vi "Teleop.vi"(10 "Match Info":T3={"Autonomous Elapsed Seconds"=0.0, "TeleOp Elapsed Seconds"=0.0, "Disabled Elapsed Seconds"=0.0, "Visited Autonomous"=FALSE, "Visited TeleOp"=FALSE, "Visited Disabled"=FALSE, "Autonomous Settings"={"Autonomous Style"=enum."Independent", "VI Refnum"=refnum}}, 11 "Call Context":T4) -> ()   [LabVIEW 2017]
doc: "This VI is called for each TeleOp packet received from the DS where the robot is not disabled. It is often used to read from the joysticks and update I/O or to update setpoints for timed control loops. It should complete and return within 20 milliseconds or it may miss DS packets."
uses:
  <vilib>/Rock Robotics/WPI/DriverStation/WPI_DriverStationDerivedRobotMode.ctl
  <vilib>/Rock Robotics/WPI/DriverStation/WPI_DriverStationMatch Info.ctl
  SwerveLibrary/Controllers.ctl
  <vilib>/Rock Robotics/WPI/Utilities/WPI_GetSetVariantRefNum.vi
  Robot Global Data.vi
  <vilib>/Rock Robotics/Network Tables/NT Write Boolean.vi
  SwerveLibrary/Huskie Swerve.lvlib
panel:
  in  "Elbow Power":dbl
  in  "Shoulder Power":dbl
  in  "Solenoids":T1
  in  "Arm Angle":T2 {"Elbow Angle (Rad)" scale=-3.14..3.14; "Shoulder Angle (Rad)" scale=-3.14..3.14}
  in  "Manual Control":bool
  # "Arm Control"
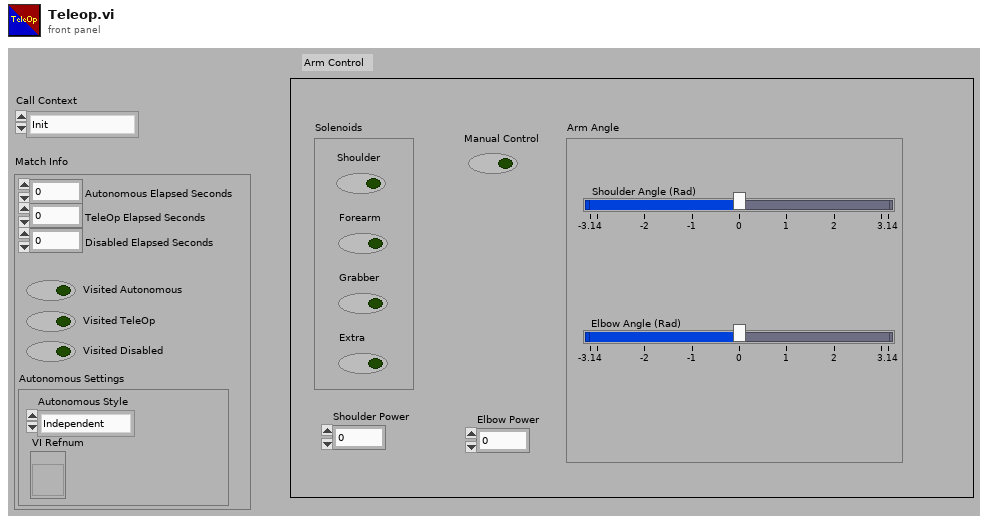
[diagram p1: front panel]
types:
  T1 = cluster{"Shoulder":bool, "Forearm":bool, "Grabber":bool, "Extra":bool}
  T2 = cluster{"Shoulder Angle (Rad)":dbl, "Elbow Angle (Rad)":dbl}
  T3 = typedef "WPI_DriverStationMatch Info.ctl" = cluster{"Autonomous Elapsed Seconds":dbl, "TeleOp Elapsed Seconds":dbl, "Disabled Elapsed Seconds":dbl, "Visited Autonomous":bool, "Visited TeleOp":bool, "Visited Disabled":bool, "Autonomous Settings":cluster{"Autonomous Style":enum16{"Iterative", "Independent"}, "VI Refnum":refnum<vi>}}
  T4 = typedef "WPI_DriverStationDerivedRobotMode.ctl" = enum16{"Init", "Execute", "Stop"}
  T5 = cluster{"X":dbl, "Y":dbl, "Z":dbl, "Climber Up":bool, "Climber Down":bool, "X Drive":bool, "Field Relative":bool, "Actuate Grabber":bool, "Inverse Drive":bool}
  T6 = typedef "Huskie Swerve.lvlib/Controllers.ctl" = enum16{"Joystick", "Buttons"}
  T7 = typedef "WPI_JoystickDevRef.ctl" = cluster{"Device":T8}
  T8 = typedef "WPI_JoystickDeviceEnum.ctl" = enum16{"USB 0", "USB 1", "USB 2", "USB 3", "USB 4", "USB 5"}
  T9 = typedef "WPI_DigitalInputDevRef.ctl" = cluster{"DevStatus":errorcluster, "DIO Channel":T10}
  T10 = typedef "FPGA_DIOChannel.ctl" = enum8{"DIO 0", "DIO 1", "DIO 2", "DIO 3", "DIO 4", "DIO 5", "DIO 6", "DIO 7", "DIO 8", "DIO 9", "DIO MXP 0", "DIO MXP 1", "DIO MXP 2", "DIO MXP 3", "DIO MXP 4", "DIO MXP 5", "DIO MXP 6", "DIO MXP 7", "DIO MXP 8", "DIO MXP 9", "DIO MXP 10", "DIO MXP 11", "DIO MXP 12", "DIO MXP 13", "DIO MXP 14", "DIO MXP 15", "SPI Port CS1", "SPI Port CS2", "SPI Port CS3", "SPI Port MISO", "SPI Port MOSI", "Invalid"}
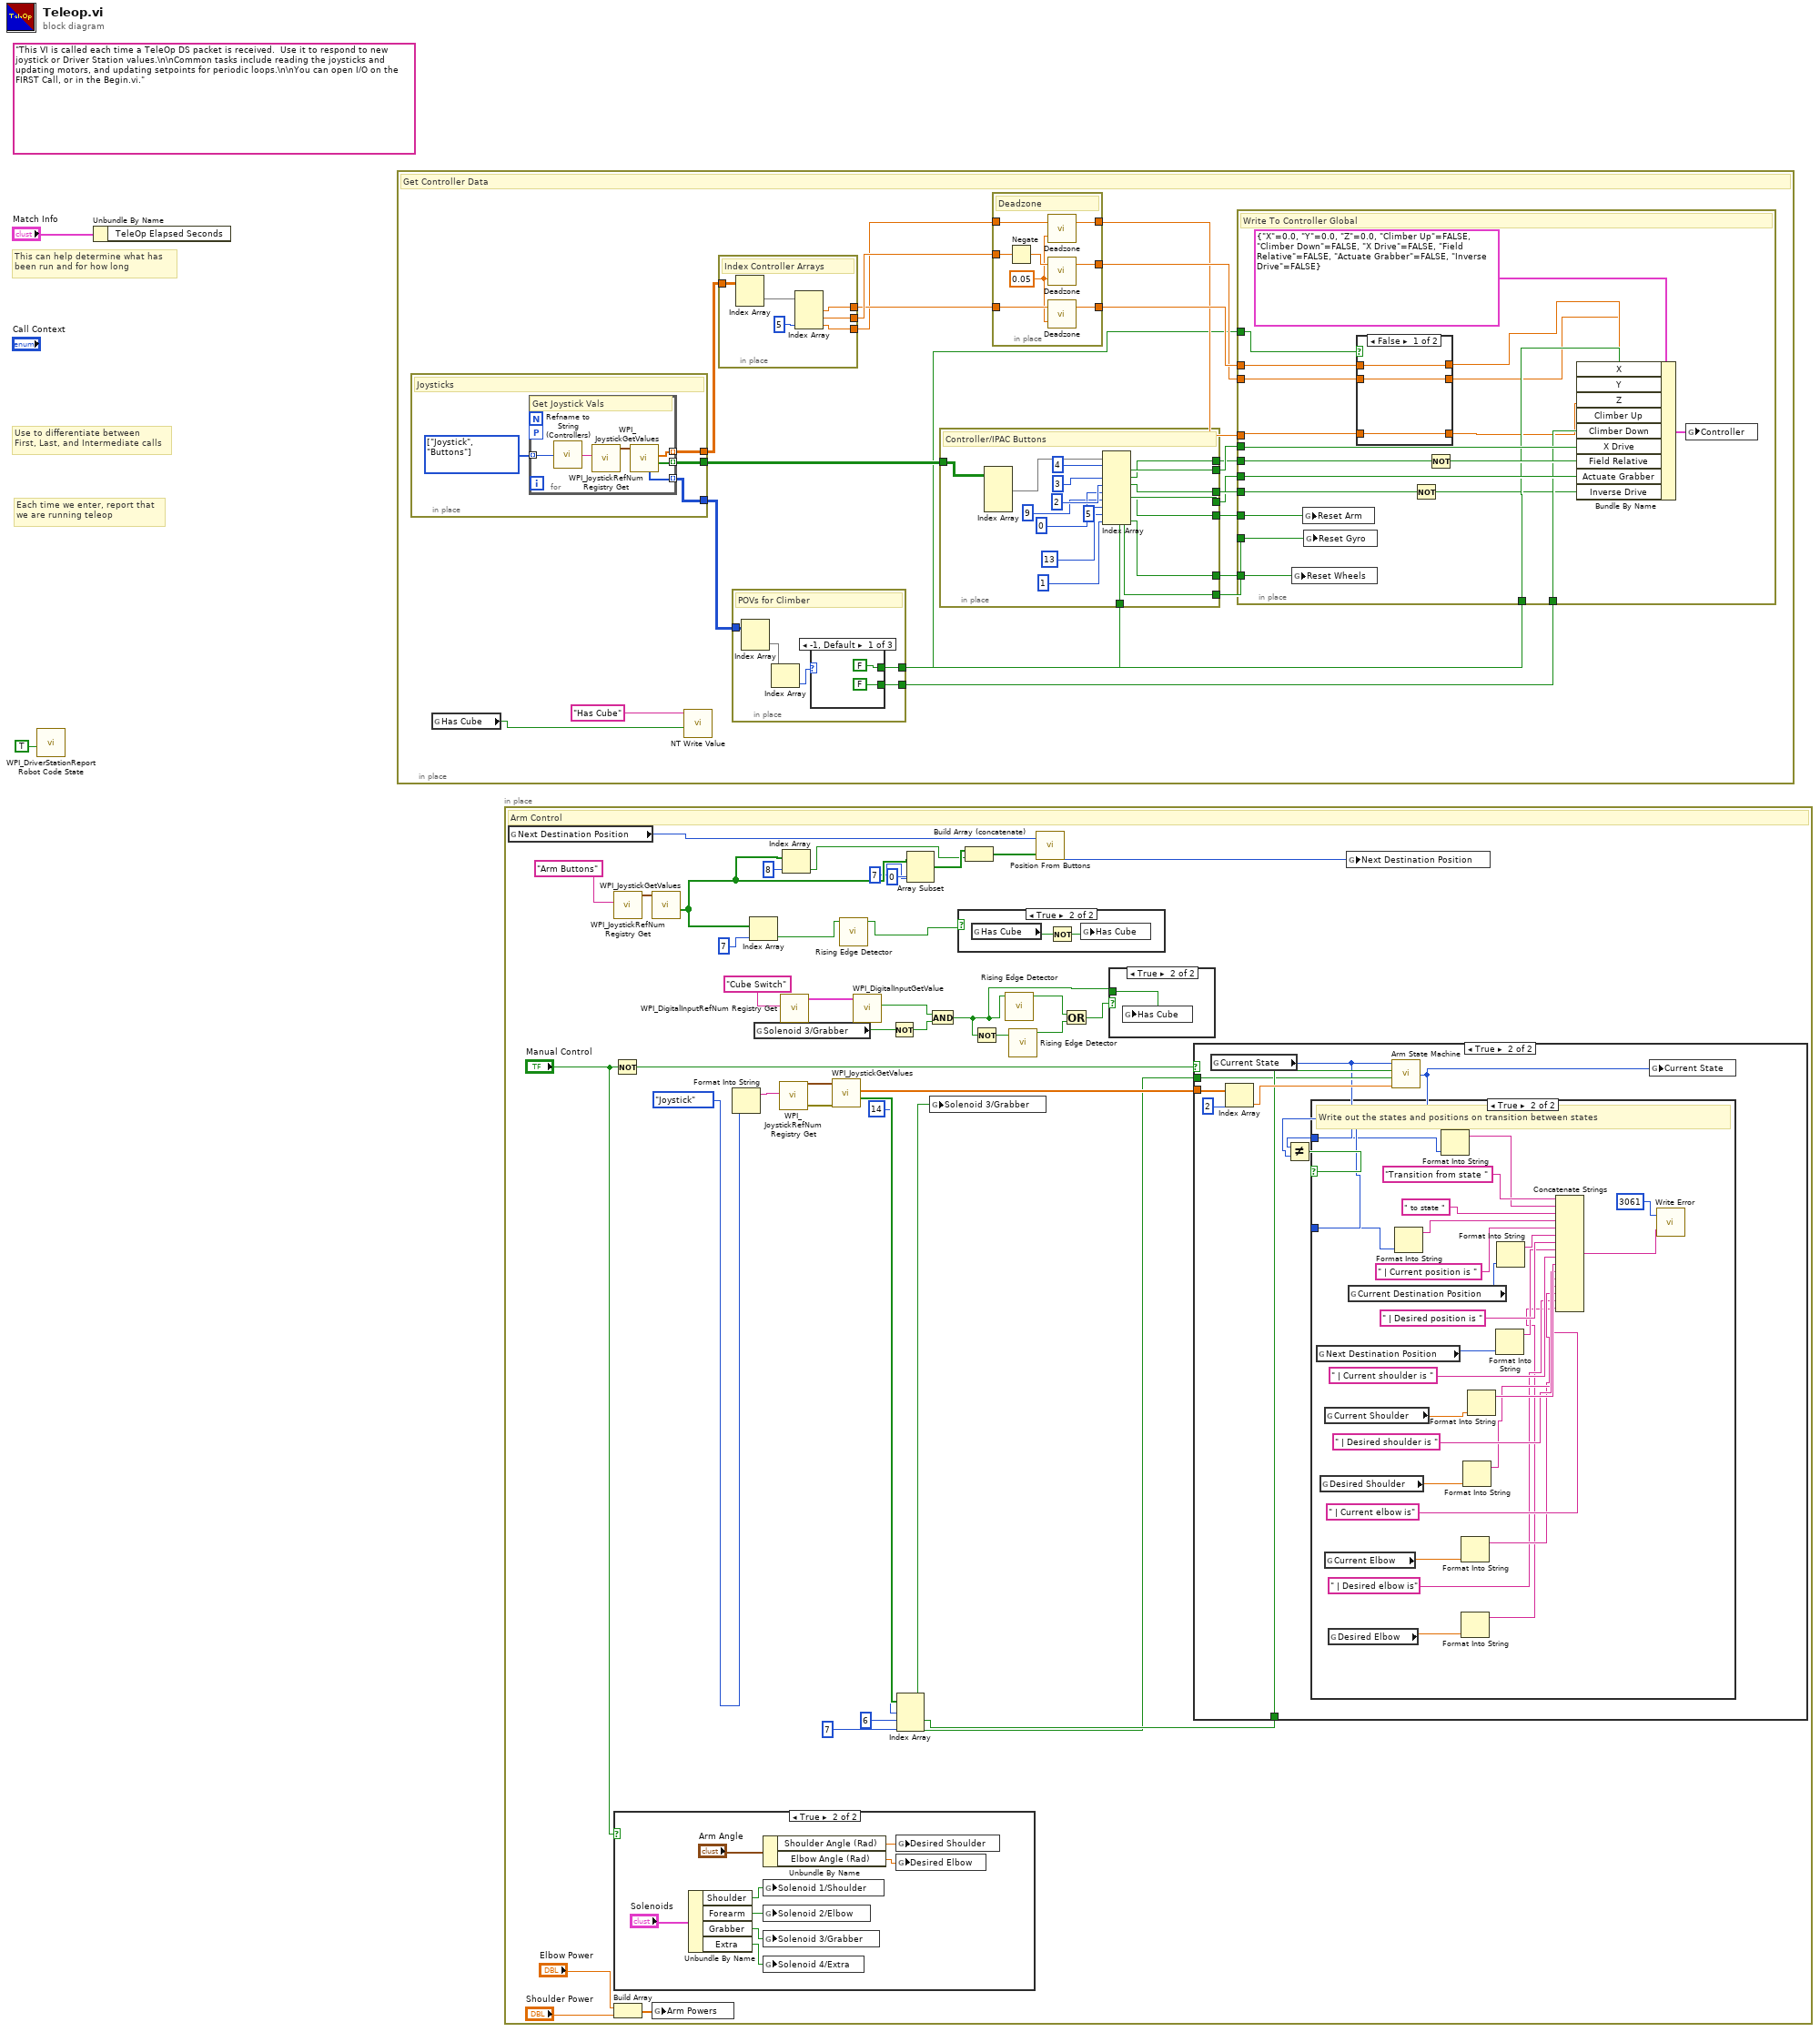
[diagram p0: block diagram]
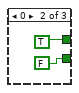
[diagram p7: hidden frame]
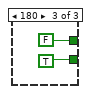
[diagram p8: hidden frame]
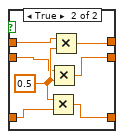
[diagram p9: hidden frame]
diagram:
  (unwired) "This VI is called each time a TeleOp DS packet is received.  Use it to respond to new joystick or Driver Station values.\n\nCommon tasks include reading the joysticks and updating motors, and updating setpoints for periodic loops.\n\nYou can open I/O on the FIRST Call, or in the Begin.vi."
  # "Each time we enter, report that\nwe are running teleop"
  # "Use to differentiate between\nFirst, Last, and Intermediate calls"
  # "This can help determine what has\nbeen run and for how long"
  n1 = call <vilib>:"WPI_DriverStationReport Robot Code State.vi"("TeleOp"=TRUE ("Autonomous")) -> ()  [unwired: 10 in, 1 out]
  n2 = Unbundle By Name("Match Info") -> ()  [unwired: 1 out]
  n3 = in-place "In Place Element Structure" {
    # "Get Controller Data"
    n4 = in-place {
      in-place-border: [w85] -> w23
      in-place-border: [w84] -> w16
      in-place-border: [w83] -> w7
      w86 = T6[] [enum."Joystick", enum."Buttons"] items=["Joystick", "Buttons"]
      # "Joysticks"
      n5 = for {
        workers-P: _ -> [_]
        tunnel: w86 -> [w92] mode=indexing
        tunnel: [w89] -> w85 mode=indexing
        tunnel: [w88] -> w84 mode=indexing
        tunnel: [w87] -> w83 mode=indexing
        # "Get Joystick Vals"
        n6 = call "Refname to String (Controllers).vi"("Enum"=w92) -> ("resulting string"=w91:string)
        n7 = call <vilib>:"WPI_JoystickRefNum Registry Get.vi"("refnum name"=w91) -> ("JoystickDevRef"=w90:T7)  [unwired: 9 in, 1 out]
        n8 = call <vilib>:"WPI_JoystickGetValues.vi"("JoystickDevRef"=w90) -> ("Buttons"=w88:bool[], "Axes"=w89:dbl[], "POVs"=w87:i16[])  [unwired: 6 in, 2 out]
      }
    }
    n9 = global read "Robot Global Data.vi" "Has Cube"() -> (w9:bool)
    n10 = call-poly <vilib>:"NT Write Value.vi"("Boolean"=w9, "Name"="Has Cube") -> ()  [unwired: 9 in, 1 out]
    n11 = in-place {
      in-place-border: w23 -> [w106]
      in-place-border: [w103] -> w22
      in-place-border: [w102] -> w21
      in-place-border: [w101] -> w17
      # "Index Controller Arrays"
      n12 = Index Array(array=w106) -> (element=w105:dbl[])  [unwired: 2 in]
      n13 = Index Array(array=w105, index #3=5) -> (element #1=w102:dbl, element #2=w103:dbl, element #3=w101:dbl)  [unwired: 2 in]
    }
    n14 = in-place "In Place Element Structure" {
      in-place-border: w7 -> [w28]
      in-place-border: [w25] -> w6
      in-place-border: [w24] -> w5
      # "POVs for Climber"
      n15 = Index Array(array=w28) -> (element=w27:i16[])  [unwired: 2 in]
      n16 = Index Array(array=w27) -> (element=w26:i16)  [unwired: 1 in]
      n17 = case shown="-1, Default" w26 {
        tunnel: [FALSE TRUE FALSE] -> w25
        tunnel: [FALSE FALSE TRUE] -> w24
        frame -1, Default {
        }
        frame 0 {
        }
        frame 180 {
        }
      }
    }
    n18 = in-place {
      in-place-border: w16 -> [w82]
      in-place-border: [w79] -> w15
      in-place-border: [w77] -> w14
      in-place-border: [w75] -> w13
      in-place-border: [w73] -> w12
      in-place-border: [w70] -> w11
      in-place-border: [w69] -> w10
      in-place-border: [w67] -> w4
      in-place-border: [w65] -> w3
      # "Controller/IPAC Buttons"
      n19 = Index Array(array=w82) -> (element #1=w81:bool[])  [unwired: 4 in, 1 out]
      n20 = Index Array(array=w81, index #1=4, index #2=3, index #3=2, index #4=0, index #5=9 ("index"), index #6=13 ("index"), index #7=5 ("index"), index #8=1 ("index")) -> (element #1=w79:bool, element #2=w77:bool, element #3=w75:bool, element #4=w73:bool, element #5=w70:bool, element #6=w69:bool, element #7=w67:bool, element #8=w65:bool)
    }
    n21 = in-place {
      in-place-border: w22 -> [w99]
      in-place-border: w21 -> [w98]
      in-place-border: [w96] -> w20
      in-place-border: [w95] -> w19
      in-place-border: [w94] -> w18
      in-place-border: w17 -> [w93]
      w97 = 0.05
      # "Deadzone"
      n22 = Negate(x=w99) -> (-x=w100:dbl)
      n23 = call "Deadzone.vi"("Deadzone"=w97, "Value"=w93) -> ("Numeric"=w94:dbl)  [unwired: 1 out]
      n24 = call "Deadzone.vi"("Deadzone"=w97, "Value"=w100) -> ("Numeric"=w95:dbl)  [unwired: 1 out]
      n25 = call "Deadzone.vi"("Deadzone"=w97, "Value"=w98) -> ("Numeric"=w96:dbl)  [unwired: 1 out]
    }
    n26 = in-place {
      in-place-border: w20 -> [w43]
      in-place-border: w19 -> [w40]
      in-place-border: w18 -> [w38]
      in-place-border: w15 -> [w52]
      in-place-border: w14 -> [w48]
      in-place-border: w13 -> [w51]
      in-place-border: w12 -> [w50]
      in-place-border: w11 -> [w47]
      in-place-border: w10 -> [w46]
      in-place-border: w6 -> [w45]
      in-place-border: w5 -> [w44]
      in-place-border: w4 -> [w41]
      in-place-border: w3 -> [w35]
      # "Write To Controller Global"
      n27 = global write "Robot Global Data.vi" "Reset Wheels"(w35) -> ()
      n28 = global write "Robot Global Data.vi" "Reset Arm"(w47) -> ()
      n29 = global write "Robot Global Data.vi" "Reset Gyro"(w46) -> ()
      n30 = case shown="False" w41 {
        tunnel: w43 -> [w57 w60]
        tunnel: [w57 w61] -> w42
        tunnel: w40 -> [w56 w63]
        tunnel: [w56 w62] -> w39
        tunnel: w38 -> [w55 w59]
        tunnel: [w55 w58] -> w37
        frame False {
        }
        frame True {
          w64 = 0.5
          n31 = Multiply(x=w64, y=w59) -> (x*y=w58:dbl)
          n32 = Multiply(x=w63, y=w64) -> (x*y=w62:dbl)
          n33 = Multiply(x=w60, y=w64) -> (x*y=w61:dbl)
        }
      }
      n34 = Not(x=w51) -> (.not. x?=w36:bool)
      n35 = Not(x=w48) -> (.not. x?=w49:bool)
      n36 = Bundle By Name(cluster=T5 {"X"=0.0, "Y"=0.0, "Z"=0.0, "Climber Up"=FALSE, "Climber Down"=FALSE, "X Drive"=FALSE, "Field Relative"=FALSE, "Actuate Grabber"=FALSE, "Inverse Drive"=FALSE}, "X"=w42, "Y"=w39, "Z"=w37, "Climber Up"=w45, "Climber Down"=w44, "X Drive"=w52, "Field Relative"=w49, "Actuate Grabber"=w50, "Inverse Drive"=w36) -> (w53:T5)
      n37 = global write "Robot Global Data.vi" "Controller"(w53) -> ()
    }
  }
  n38 = in-place "In Place Element Structure" {
    # "Arm Control"
    n39 = global read "Robot Global Data.vi" "Next Destination Position"() -> (w127:i32)
    n40 = Not(x="Manual Control") -> (.not. x?=w144:bool)
    n41 = call <vilib>:"WPI_JoystickRefNum Registry Get.vi"("refnum name"="Arm Buttons") -> ("JoystickDevRef"=w146:T7)  [unwired: 9 in, 1 out]
    n42 = case shown="True" "Manual Control" {
      frame False {
      }
      frame True {
        n43 = Unbundle By Name("Solenoids") -> ("Shoulder"=w189:bool, "Forearm"=w190:bool, "Grabber"=w191:bool, "Extra"=w192:bool)
        n44 = Unbundle By Name("Arm Angle") -> ("Shoulder Angle (Rad)"=w187:dbl, "Elbow Angle (Rad)"=w186:dbl)
        n45 = global write "Robot Global Data.vi" "Solenoid 1/Shoulder"(w189) -> ()
        n46 = global write "Robot Global Data.vi" "Solenoid 2/Elbow"(w190) -> ()
        n47 = global write "Robot Global Data.vi" "Solenoid 3/Grabber"(w191) -> ()
        n48 = global write "Robot Global Data.vi" "Solenoid 4/Extra"(w192) -> ()
        n49 = global write "Robot Global Data.vi" "Desired Shoulder"(w187) -> ()
        n50 = global write "Robot Global Data.vi" "Desired Elbow"(w186) -> ()
      }
    }
    n51 = Build Array("Elbow Power", "Shoulder Power") -> (w141:dbl[])
    n52 = call <vilib>:"WPI_JoystickGetValues.vi"("JoystickDevRef"=w146) -> ("Buttons"=w124:bool[])  [unwired: 6 in, 4 out]
    n53 = global write "Robot Global Data.vi" "Arm Powers"(w141) -> ()
    n54 = Format Into String(Controllers."Joystick" ("Enum")) -> (resulting string=w138:string)  [unwired: 3 in, 1 out]
    n55 = Index Array(array=w124, index=7) -> (element=w113:bool)
    n56 = global read "Robot Global Data.vi" "Solenoid 3/Grabber"() -> (w117:bool)
    n57 = call <vilib>:"WPI_JoystickRefNum Registry Get.vi"("refnum name"=w138) -> ("error out"=w136:errorcluster, "JoystickDevRef"=w137:T7)  [unwired: 9 in]
    n58 = call <vilib>:"WPI_DigitalInputRefNum Registry Get.vi"("refnum name"="Cube Switch") -> ("DigitalInputDevRef"=w116:T9)  [unwired: 9 in, 1 out]
    n59 = Index Array(array=w124, index=8) -> (element=w122:bool)
    n60 = call <vilib>:"WPI_JoystickGetValues.vi"("error in (no error)"=w136, "JoystickDevRef"=w137) -> ("Buttons"=w135:bool[], "Axes"=w133:dbl[])  [unwired: 5 in, 3 out]
    n61 = call "Rising Edge Detector.vi"("Input"=w113) -> ("Rising edge?"=w112:bool)  [unwired: 10 in]
    n62 = call <vilib>:"WPI_DigitalInputGetValue.vi"("DigitalInputDevRef"=w116) -> ("Value"=w119:bool)  [unwired: 8 in, 2 out]
    n63 = Not(x=w117) -> (.not. x?=w118:bool)
    n64 = Index Array(array=w135, index #1=14 ("index"), index #2=6 ("index"), index #3=7 ("index")) -> (element #1=w134:bool, element #2=w131:bool, element #3=w128:bool)
    n65 = Array Subset(array=w124, index=0, length=7) -> (w123:bool[])
    n66 = And(x=w119, y=w118) -> (x .and. y?=w107:bool)
    n67 = global write "Robot Global Data.vi" "Solenoid 3/Grabber"(w134) -> ()
    n68 = case shown="True" w112 {
      frame False {
      }
      frame True {
        n69 = global read "Robot Global Data.vi" "Has Cube"() -> (w149:bool)
        n70 = Not(x=w149) -> (.not. x?=w150:bool)
        n71 = global write "Robot Global Data.vi" "Has Cube"(w150) -> ()
      }
    }
    n72 = Build Array (concatenate)(w123, w122) -> (w121:bool[])
    n73 = Not(x=w107) -> (.not. x?=w111:bool)
    n74 = call "Rising Edge Detector.vi"("Input"=w107) -> ("Rising edge?"=w110:bool)  [unwired: 10 in]
    n75 = call "Rising Edge Detector.vi"("Input"=w111) -> ("Rising edge?"=w109:bool)  [unwired: 10 in]
    n76 = call "Position From Buttons.vi"("Buttons"=w121, "Current Position"=w127) -> ("Desired Position"=w147:i32)
    n77 = Or(x=w110, y=w109) -> (x .or. y?=w108:bool)
    n78 = case shown="True" w108 {
      tunnel: w107 -> [_ w148]
      frame False {
      }
      frame True {
        n79 = global write "Robot Global Data.vi" "Has Cube"(w148) -> ()
      }
    }
    n80 = case shown="True" w144 {
      tunnel: w133 -> [_ w158]
      tunnel: w131 -> [_ w155]
      tunnel: w128 -> [_ w154]
      frame False {
      }
      frame True {
        n81 = global read "Robot Global Data.vi" "Current State"() -> (w152:i32)
        n82 = Index Array(array=w158, index=2) -> (element=w156:dbl)
        n83 = call "Arm State Machine.vi"("Delta Angle"=w156, "Shoulder Control"=w154, "Forearm Control"=w155, "State"=w152) -> ("Next State"=w151:i32)
        n84 = Not Equal?(x=w152, y=w151) -> (x != y?=w153:bool)
        n85 = case shown="True" w153 {
          tunnel: w152 -> [_ w183]
          tunnel: w151 -> [_ w180]
          frame False {
          }
          frame True {
            # "Write out the states and positions on transition between states"
            n86 = global read "Robot Global Data.vi" "Next Destination Position"() -> (w174:i32)
            n87 = global read "Robot Global Data.vi" "Desired Shoulder"() -> (w165:dbl)
            n88 = global read "Robot Global Data.vi" "Current Shoulder"() -> (w169:dbl)
            n89 = global read "Robot Global Data.vi" "Current Elbow"() -> (w166:dbl)
            n90 = global read "Robot Global Data.vi" "Desired Elbow"() -> (w167:dbl)
            n91 = global read "Robot Global Data.vi" "Current Destination Position"() -> (w176:i32)
            n92 = Format Into String(w180) -> (resulting string=w179:string)  [unwired: 3 in, 1 out]
            n93 = Format Into String(w183) -> (resulting string=w182:string)  [unwired: 3 in, 1 out]
            n94 = Format Into String(w166) -> (resulting string=w161:string)  [unwired: 3 in, 1 out]
            n95 = Format Into String(w167) -> (resulting string=w159:string)  [unwired: 3 in, 1 out]
            n96 = Format Into String(w165) -> (resulting string=w163:string)  [unwired: 3 in, 1 out]
            n97 = Format Into String(w169) -> (resulting string=w168:string)  [unwired: 3 in, 1 out]
            n98 = Format Into String(w174) -> (resulting string=w173:string)  [unwired: 3 in, 1 out]
            n99 = Format Into String(w176) -> (resulting string=w177:string)  [unwired: 3 in, 1 out]
            n100 = Concatenate Strings("Transition from state ", w182, " to state ", w179, " | Current position is ", w177, " | Desired position is ", w173, " | Current shoulder is ", w168, " | Desired shoulder is ", w163, " | Current elbow is", w161, " | Desired elbow is", w159) -> (w172:string)
            n101 = call "Write Error.vi"("Message To Write"=w172, "Error Code"=3061) -> ()  [unwired: 1 out]
          }
        }
        n102 = global write "Robot Global Data.vi" "Current State"(w151) -> ()
      }
    }
    n103 = global write "Robot Global Data.vi" "Next Destination Position"(w147) -> ()
  }
